vi "Autonomous Independent.vi"   [LabVIEW 2013]
doc: "This VI is called when autonomous begins, and will automatically be terminated when autonomous ends. You can carry out timed or sensor driven robot movement independently without needing to return to the caller."
uses:
  <vilib>/Rock Robotics/WPI/Solenoid/WPI_SolenoidValue.ctl
  Robot Global Data.vi
  <vilib>/Rock Robotics/WPI/Solenoid/WPI_SolenoidSetEnum.vi
  <vilib>/Rock Robotics/WPI/RobotDrive/WPI_RobotDriveArcadeDrive_Standard(NoSaturation).vi
  <vilib>/Rock Robotics/WPI/RobotDrive/WPI_RobotDriveGetSetRefNum.vi
  <vilib>/Rock Robotics/WPI/Joystick/WPI_JoystickGetSetRefNum.vi
panel:
  # "Be sure to right-click and choose Data Operations>>Make Current Value default if you want to save the array values with the VI"
types:
  T1 = typedef "WPI_JoystickDevRef.ctl" = cluster{"Device":T2}
  T2 = typedef "WPI_JoystickDeviceEnum.ctl" = enum16{"USB 1", "USB 2", "USB 3", "USB 4", "Kinect 1", "Kinect 2"}
  T3 = cluster{"axis 1 (x)":dbl, "axis 2 (y)":dbl, "axis 3 (throttle)":dbl, "axis 4":dbl, "axis 5":dbl, "axis 6":dbl}
  T4 = typedef "WPI_SolenoidValue.ctl" = enum16{"Off", "On", "Forward", "Reverse"}
  T5 = typedef "WPI_DigitalInputDevRef.ctl" = cluster{"DevStatus":errorcluster, "DIO Channel":T6, "Digital Module":T7}
  T6 = typedef "FPGA_DIOChannel.ctl" = enum8{"DIO 1", "DIO 2", "DIO 3", "DIO 4", "DIO 5", "DIO 6", "DIO 7", "DIO 8", "DIO 9", "DIO 10", "DIO 11", "DIO 12", "DIO 13", "DIO 14", "Invalid"}
  T7 = typedef "FPGA_TypedefDigitalModule.ctl" = enum16{"Digital Module 1", "Digital Module 2"}
  T8 = typedef "WPI_SolenoidDevRef.ctl" = cluster{"DevStatus":errorcluster, "Solenoid Module":T9, "Forward Solenoid Channel":T10, "Reverse Solenoid Channel":T10}
  T9 = typedef "FPGA_TypedefSolenoidModule.ctl" = enum16{"Solenoid Module 1", "Solenoid Module 2"}
  T10 = typedef "WPI_SolenoidChannel.ctl" = enum8{"Solenoid 1", "Solenoid 2", "Solenoid 3", "Solenoid 4", "Solenoid 5", "Solenoid 6", "Solenoid 7", "Solenoid 8", "Invalid"}
  T11 = typedef "WPI_RobotDriveDevRef.ctl" = cluster{"DevStatus":errorcluster, "Motors[]":T12[], "Square Inputs":bool, "Max Output":dbl, "Isochronous":bool}
  T12 = typedef "WPI_MotorControlDeviceRef.ctl" = cluster{"DeviceStatus":errorcluster, "Type":enum16{"PWM", "CAN"}, "PWM":cluster{"Digital Module":T7, "PWM Channel":T13, "DeadBand":T14}, "CAN":cluster{"Device Number":u8, "Control Mode":T15, "Semaphore":T16, "Max Vout":dbl}, "Invert":bool, "TransformRef":T17, "InvTransformRef":T17}
  T13 = typedef "FPGA_DIOPWMChannel.ctl" = enum8{"PWM 1", "PWM 2", "PWM 3", "PWM 4", "PWM 5", "PWM 6", "PWM 7", "PWM 8", "PWM 9", "PWM 10", "Invalid"}
  T14 = typedef "WPI_PWMDeadband.ctl" = cluster{"Name":string, "maxPositivePwm":i32, "minPositivePwm":i32, "centerPwm":i32, "maxNegativePwm":i32, "minNegativePwm":i32, "angularRange":u16}
  T15 = typedef "WPI_CANJaguar_ControlMode.ctl" = enum8{"Percent VBus", "Current", "Speed", "Position", "Voltage"}
  T16 = typedef "Semaphore RefNum" = refnum<k1>
  T17 = typedef "WPI_PWMTransform_ConPane.ctl" = refnum<vi>
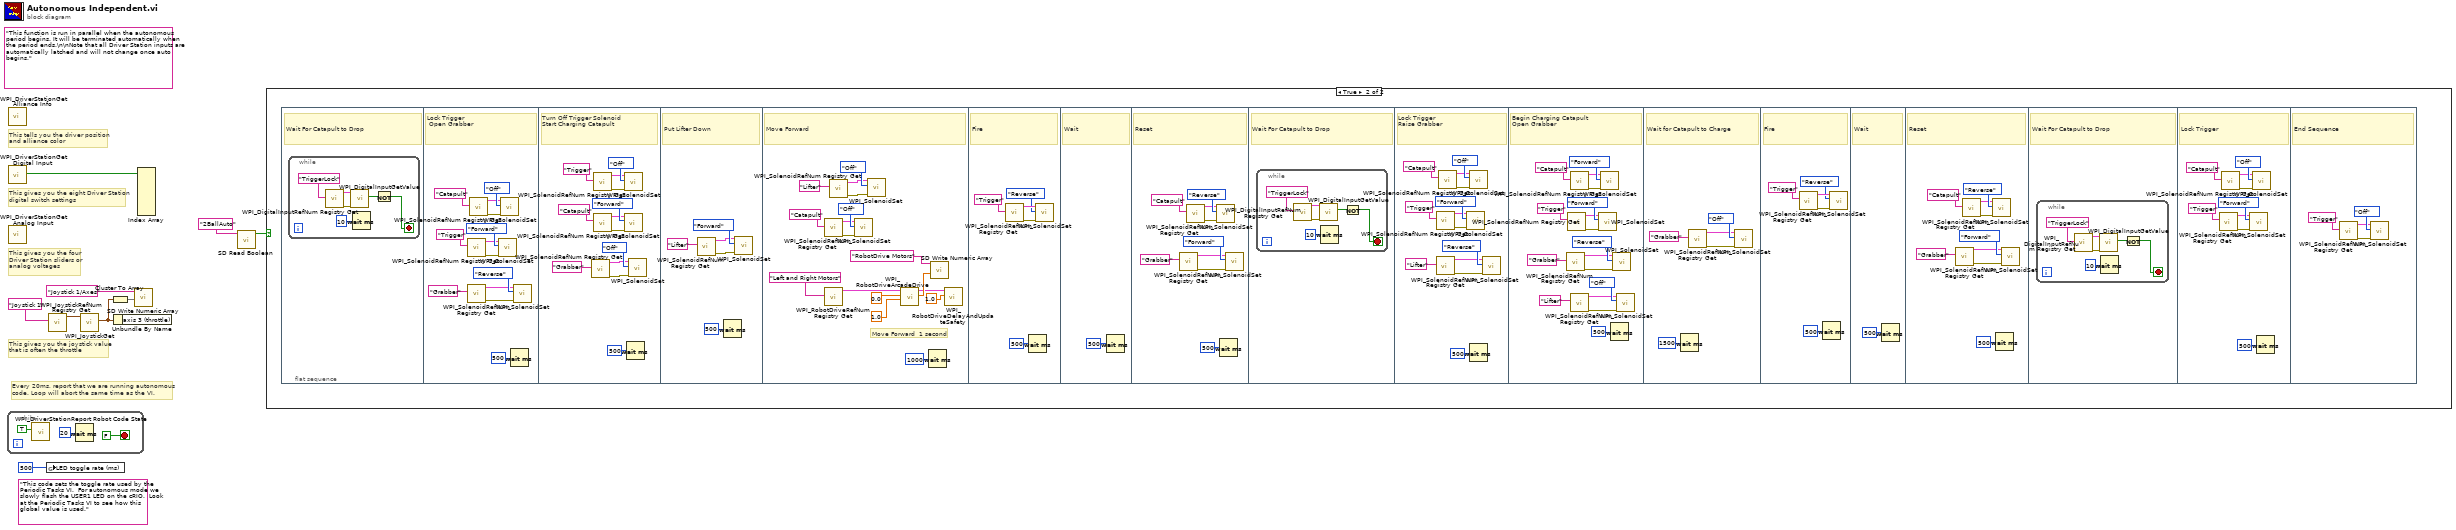
[diagram p0: block diagram]
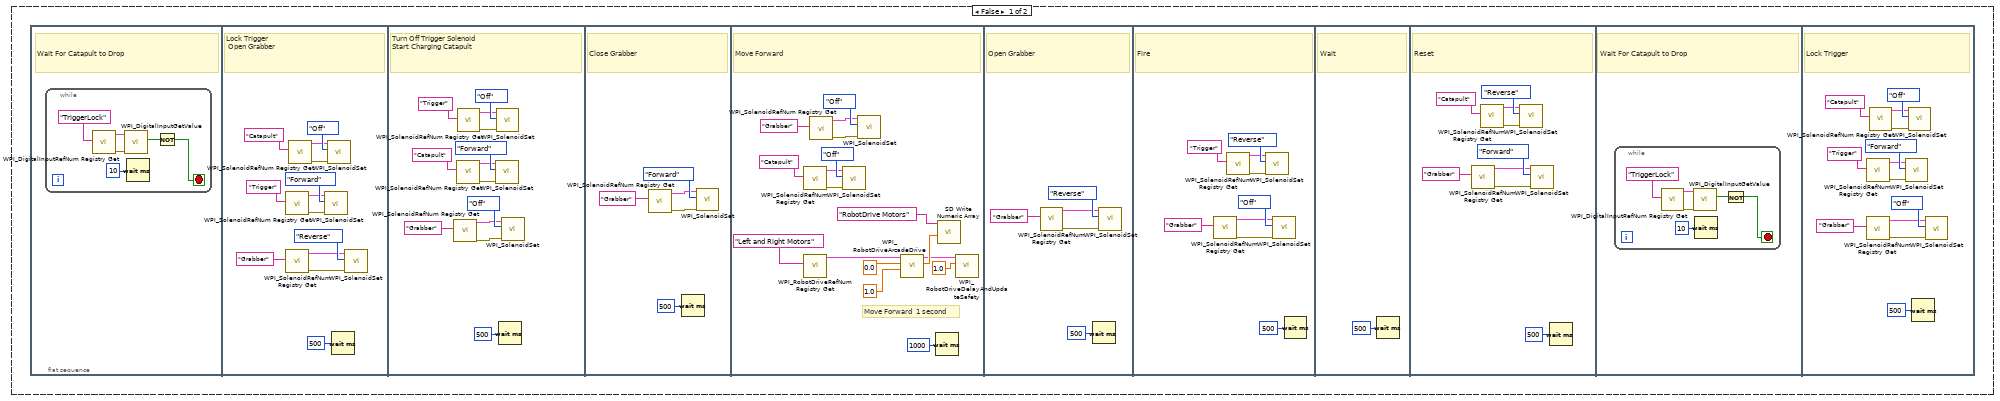
[diagram p2: hidden frame]
diagram:
  (unwired) "This code sets the toggle rate used by the Periodic Tasks VI.  For autonomous mode we slowly flash the USER1 LED on the cRIO.  Look at the Periodic Tasks VI to see how this global value is used."
  (unwired) "This function is run in parallel when the autonomous period begins. It will be terminated automatically when the period ends.\n\nNote that all Driver Station inputs are automatically latched and will not change once auto begins."
  # "Every 20ms, report that we are running autonomous\ncode. Loop will abort the same time as the VI."
  # "This gives you the joystick value\nthat is often the throttle"
  # "This tells you the driver position\nand alliance color"
  # "This gives you the eight Driver Station\ndigital switch settings"
  # "This gives you the four\nDriver Station sliders or\nanalog voltages"
  n1 = while {
    stop <- FALSE stop-if-true
    n2 = call <vilib>:"WPI_DriverStationReport Robot Code State.vi"("Autonomous"=TRUE) -> ()  [unwired: 10 in, 1 out]
    n3 = Wait (ms)(milliseconds to wait=u32 20) -> ()  [unwired: 1 out]
  }
  n4 = call <vilib>:"WPI_DriverStationGet Alliance Info.vi"() -> ()  [unwired: 12 out]
  n5 = call <vilib>:"WPI_DriverStationGet Digital Input.vi"() -> ("Driver Station Digital Input (1-8)"=w9:bool[])  [unwired: 11 out]
  n6 = call <vilib>:"WPI_DriverStationGet Analog Input.vi"() -> ()  [unwired: 12 out]
  n7 = global write "Robot Global Data.vi" "LED toggle rate (ms)"(u32 500 ("LED ms toggle rate")) -> ()
  n8 = call <vilib>:"WPI_JoystickRefNum Registry Get.vi"("refnum name"="Joystick 1") -> ("JoystickDevRef"=w7:T1)  [unwired: 1 in, 9 out]
  n9 = call <vilib>:"WPI_JoystickGet.vi"("JoystickDevRef"=w7) -> ("Axes"=w4:T3)  [unwired: 1 in, 5 out]
  n10 = Cluster To Array(cluster=w4) -> (array=w5:dbl[])
  n11 = Unbundle By Name(w4) -> ()  [unwired: 1 out]
  n12 = call <vilib>:"SD Write Numeric Array.vi"("Numeric Array"=w5, "Name"="Joystick 1/Axes") -> ()  [unwired: 8 in, 2 out]
  n13 = Index Array(array=w9) -> ()  [unwired: 8 in, 8 out]
  n14 = call <vilib>:"SD Read Boolean.vi"("Name"="2BallAuto") -> ("Boolean"=w1:bool)  [unwired: 8 in, 2 out]
  n15 = case shown="True" w1 {
    frame False {
      n16 = flat-sequence {
        frame #0 {
          # "Wait For Catapult to Drop"
          n17 = while {
            stop <- w14 stop-if-true
            n18 = call <vilib>:"WPI_DigitalInputRefNum Registry Get.vi"("refnum name"="TriggerLock") -> ("error out"=w15:errorcluster, "DigitalInputDevRef"=w16:T5)  [unwired: 9 in]
            n19 = call <vilib>:"WPI_DigitalInputGetValue.vi"("error in (no error)"=w15, "DigitalInputDevRef"=w16) -> ("Value"=w17:bool)  [unwired: 7 in, 2 out]
            n20 = Wait (ms)(milliseconds to wait=u32 10) -> ()  [unwired: 1 out]
            n21 = Not(x=w17) -> (.not. x?=w14:bool)
          }
        }
        frame #1 {
          # "Lock Trigger\n Open Grabber"
          n22 = call <vilib>:"WPI_SolenoidRefNum Registry Get.vi"("refnum name"="Trigger") -> ("error out"=w24:errorcluster, "SolenoidDevRef"=w25:T8)  [unwired: 9 in]
          n23 = call <vilib>:"WPI_SolenoidRefNum Registry Get.vi"("refnum name"="Grabber") -> ("error out"=w20:errorcluster, "SolenoidDevRef"=w21:T8)  [unwired: 9 in]
          n24 = call <vilib>:"WPI_SolenoidRefNum Registry Get.vi"("refnum name"="Catapult") -> ("error out"=w28:errorcluster, "SolenoidDevRef"=w29:T8)  [unwired: 9 in]
          n25 = call-poly <vilib>:"WPI_SolenoidSet.vi"("error in (no error)"=w24, "Value"=WPI_SolenoidValue."Forward", "SolenoidDevRef"=w25) -> ()  [unwired: 7 in, 2 out]
          n26 = call-poly <vilib>:"WPI_SolenoidSet.vi"("error in (no error)"=w28, "Value"=WPI_SolenoidValue."Off", "SolenoidDevRef"=w29) -> ()  [unwired: 7 in, 2 out]
          n27 = Wait (ms)(milliseconds to wait=u32 500) -> ()  [unwired: 1 out]
          n28 = call-poly <vilib>:"WPI_SolenoidSet.vi"("error in (no error)"=w20, "Value"=WPI_SolenoidValue."Reverse", "SolenoidDevRef"=w21) -> ()  [unwired: 7 in, 2 out]
        }
        frame #2 {
          # "Turn Off Trigger Solenoid\nStart Charging Catapult"
          n29 = call <vilib>:"WPI_SolenoidRefNum Registry Get.vi"("refnum name"="Grabber") -> ("error out"=w33:errorcluster, "SolenoidDevRef"=w34:T8)  [unwired: 9 in]
          n30 = call <vilib>:"WPI_SolenoidRefNum Registry Get.vi"("refnum name"="Catapult") -> ("error out"=w38:errorcluster, "SolenoidDevRef"=w39:T8)  [unwired: 9 in]
          n31 = call <vilib>:"WPI_SolenoidRefNum Registry Get.vi"("refnum name"="Trigger") -> ("error out"=w42:errorcluster, "SolenoidDevRef"=w43:T8)  [unwired: 9 in]
          n32 = call-poly <vilib>:"WPI_SolenoidSet.vi"("error in (no error)"=w38, "Value"=WPI_SolenoidValue."Forward", "SolenoidDevRef"=w39) -> ()  [unwired: 7 in, 2 out]
          n33 = call-poly <vilib>:"WPI_SolenoidSet.vi"("error in (no error)"=w42, "Value"=WPI_SolenoidValue."Off", "SolenoidDevRef"=w43) -> ()  [unwired: 7 in, 2 out]
          n34 = Wait (ms)(milliseconds to wait=u32 500) -> ()  [unwired: 1 out]
          n35 = call-poly <vilib>:"WPI_SolenoidSet.vi"("error in (no error)"=w33, "Value"=WPI_SolenoidValue."Off", "SolenoidDevRef"=w34) -> ()  [unwired: 7 in, 2 out]
        }
        frame #3 {
          # "Close Grabber"
          n36 = call <vilib>:"WPI_SolenoidRefNum Registry Get.vi"("refnum name"="Grabber") -> ("error out"=w46:errorcluster, "SolenoidDevRef"=w47:T8)  [unwired: 9 in]
          n37 = Wait (ms)(milliseconds to wait=u32 500) -> ()  [unwired: 1 out]
          n38 = call-poly <vilib>:"WPI_SolenoidSet.vi"("error in (no error)"=w46, "Value"=WPI_SolenoidValue."Forward", "SolenoidDevRef"=w47) -> ()  [unwired: 7 in, 2 out]
        }
        frame #4 {
          # "Move Forward  1 second"
          # "Move Forward"
          n39 = call <vilib>:"WPI_SolenoidRefNum Registry Get.vi"("refnum name"="Catapult") -> ("error out"=w51:errorcluster, "SolenoidDevRef"=w52:T8)  [unwired: 9 in]
          n40 = call <vilib>:"WPI_RobotDriveRefNum Registry Get.vi"("refnum name"="Left and Right Motors") -> ("RobotDriveDevRef"=w64:T11)  [unwired: 1 in, 9 out]
          n41 = call <vilib>:"WPI_SolenoidRefNum Registry Get.vi"("refnum name"="Grabber") -> ("error out"=w55:errorcluster, "SolenoidDevRef"=w56:T8)  [unwired: 9 in]
          n42 = call-poly <vilib>:"WPI_SolenoidSet.vi"("error in (no error)"=w51, "Value"=WPI_SolenoidValue."Off", "SolenoidDevRef"=w52) -> ()  [unwired: 7 in, 2 out]
          n43 = call-poly <vilib>:"WPI_SolenoidSet.vi"("error in (no error)"=w55, "Value"=WPI_SolenoidValue."Off", "SolenoidDevRef"=w56) -> ()  [unwired: 7 in, 2 out]
          n44 = call-poly <vilib>:"WPI_RobotDriveArcadeDrive.vi"("Y axis value"=1.0 ("X axis value"), "X axis value"=0.0, "RobotDriveDevRef"=w64) -> ("Motor Values"=w65:dbl[], "RobotDriveDevRef"=w61:T11)  [unwired: 1 in, 6 out]
          n45 = Wait (ms)(milliseconds to wait=u32 1000) -> ()  [unwired: 1 out]
          n46 = call <vilib>:"SD Write Numeric Array.vi"("Numeric Array"=w65, "Name"="RobotDrive Motors") -> ()  [unwired: 8 in, 2 out]
          n47 = call <vilib>:"WPI_RobotDriveDelayAndUpdateSafety.vi"("Delay (s)"=1.0, "RobotDriveDevRef"=w61) -> ()  [unwired: 8 in, 2 out]
        }
        frame #5 {
          # "Open Grabber"
          n48 = call <vilib>:"WPI_SolenoidRefNum Registry Get.vi"("refnum name"="Grabber") -> ("error out"=w69:errorcluster, "SolenoidDevRef"=w70:T8)  [unwired: 9 in]
          n49 = Wait (ms)(milliseconds to wait=u32 500) -> ()  [unwired: 1 out]
          n50 = call-poly <vilib>:"WPI_SolenoidSet.vi"("error in (no error)"=w69, "Value"=WPI_SolenoidValue."Reverse", "SolenoidDevRef"=w70) -> ()  [unwired: 7 in, 2 out]
        }
        frame #6 {
          # "Fire"
          n51 = call <vilib>:"WPI_SolenoidRefNum Registry Get.vi"("refnum name"="Grabber") -> ("error out"=w73:errorcluster, "SolenoidDevRef"=w74:T8)  [unwired: 9 in]
          n52 = call <vilib>:"WPI_SolenoidRefNum Registry Get.vi"("refnum name"="Trigger") -> ("error out"=w77:errorcluster, "SolenoidDevRef"=w78:T8)  [unwired: 9 in]
          n53 = call-poly <vilib>:"WPI_SolenoidSet.vi"("error in (no error)"=w77, "Value"=WPI_SolenoidValue."Reverse", "SolenoidDevRef"=w78) -> ()  [unwired: 7 in, 2 out]
          n54 = call-poly <vilib>:"WPI_SolenoidSet.vi"("error in (no error)"=w73, "Value"=WPI_SolenoidValue."Off", "SolenoidDevRef"=w74) -> ()  [unwired: 7 in, 2 out]
          n55 = Wait (ms)(milliseconds to wait=u32 500) -> ()  [unwired: 1 out]
        }
        frame #7 {
          # "Wait"
          n56 = Wait (ms)(milliseconds to wait=u32 500) -> ()  [unwired: 1 out]
        }
        frame #8 {
          # "Reset"
          n57 = call <vilib>:"WPI_SolenoidRefNum Registry Get.vi"("refnum name"="Grabber") -> ("error out"=w88:errorcluster, "SolenoidDevRef"=w89:T8)  [unwired: 9 in]
          n58 = call <vilib>:"WPI_SolenoidRefNum Registry Get.vi"("refnum name"="Catapult") -> ("error out"=w84:errorcluster, "SolenoidDevRef"=w85:T8)  [unwired: 9 in]
          n59 = call-poly <vilib>:"WPI_SolenoidSet.vi"("error in (no error)"=w84, "Value"=WPI_SolenoidValue."Reverse", "SolenoidDevRef"=w85) -> ()  [unwired: 7 in, 2 out]
          n60 = call-poly <vilib>:"WPI_SolenoidSet.vi"("error in (no error)"=w88, "Value"=WPI_SolenoidValue."Forward", "SolenoidDevRef"=w89) -> ()  [unwired: 7 in, 2 out]
          n61 = Wait (ms)(milliseconds to wait=u32 500) -> ()  [unwired: 1 out]
        }
        frame #9 {
          # "Wait For Catapult to Drop"
          n62 = while {
            stop <- w92 stop-if-true
            n63 = call <vilib>:"WPI_DigitalInputRefNum Registry Get.vi"("refnum name"="TriggerLock") -> ("error out"=w93:errorcluster, "DigitalInputDevRef"=w94:T5)  [unwired: 9 in]
            n64 = call <vilib>:"WPI_DigitalInputGetValue.vi"("error in (no error)"=w93, "DigitalInputDevRef"=w94) -> ("Value"=w95:bool)  [unwired: 7 in, 2 out]
            n65 = Wait (ms)(milliseconds to wait=u32 10) -> ()  [unwired: 1 out]
            n66 = Not(x=w95) -> (.not. x?=w92:bool)
          }
        }
        frame #10 {
          # "Lock Trigger"
          n67 = call <vilib>:"WPI_SolenoidRefNum Registry Get.vi"("refnum name"="Trigger") -> ("error out"=w102:errorcluster, "SolenoidDevRef"=w103:T8)  [unwired: 9 in]
          n68 = call <vilib>:"WPI_SolenoidRefNum Registry Get.vi"("refnum name"="Grabber") -> ("error out"=w98:errorcluster, "SolenoidDevRef"=w99:T8)  [unwired: 9 in]
          n69 = call <vilib>:"WPI_SolenoidRefNum Registry Get.vi"("refnum name"="Catapult") -> ("error out"=w106:errorcluster, "SolenoidDevRef"=w107:T8)  [unwired: 9 in]
          n70 = call-poly <vilib>:"WPI_SolenoidSet.vi"("error in (no error)"=w102, "Value"=WPI_SolenoidValue."Forward", "SolenoidDevRef"=w103) -> ()  [unwired: 7 in, 2 out]
          n71 = call-poly <vilib>:"WPI_SolenoidSet.vi"("error in (no error)"=w106, "Value"=WPI_SolenoidValue."Off", "SolenoidDevRef"=w107) -> ()  [unwired: 7 in, 2 out]
          n72 = Wait (ms)(milliseconds to wait=u32 500) -> ()  [unwired: 1 out]
          n73 = call-poly <vilib>:"WPI_SolenoidSet.vi"("error in (no error)"=w98, "Value"=WPI_SolenoidValue."Off", "SolenoidDevRef"=w99) -> ()  [unwired: 7 in, 2 out]
        }
      }
    }
    frame True {
      n74 = flat-sequence {
        frame #0 {
          # "Wait For Catapult to Drop"
          n75 = while {
            stop <- w111 stop-if-true
            n76 = call <vilib>:"WPI_DigitalInputRefNum Registry Get.vi"("refnum name"="TriggerLock") -> ("error out"=w112:errorcluster, "DigitalInputDevRef"=w113:T5)  [unwired: 9 in]
            n77 = call <vilib>:"WPI_DigitalInputGetValue.vi"("error in (no error)"=w112, "DigitalInputDevRef"=w113) -> ("Value"=w114:bool)  [unwired: 7 in, 2 out]
            n78 = Wait (ms)(milliseconds to wait=u32 10) -> ()  [unwired: 1 out]
            n79 = Not(x=w114) -> (.not. x?=w111:bool)
          }
        }
        frame #1 {
          # "Lock Trigger\n Open Grabber"
          n80 = call <vilib>:"WPI_SolenoidRefNum Registry Get.vi"("refnum name"="Trigger") -> ("error out"=w121:errorcluster, "SolenoidDevRef"=w122:T8)  [unwired: 9 in]
          n81 = call <vilib>:"WPI_SolenoidRefNum Registry Get.vi"("refnum name"="Grabber") -> ("error out"=w117:errorcluster, "SolenoidDevRef"=w118:T8)  [unwired: 9 in]
          n82 = call <vilib>:"WPI_SolenoidRefNum Registry Get.vi"("refnum name"="Catapult") -> ("error out"=w125:errorcluster, "SolenoidDevRef"=w126:T8)  [unwired: 9 in]
          n83 = call-poly <vilib>:"WPI_SolenoidSet.vi"("error in (no error)"=w121, "Value"=WPI_SolenoidValue."Forward", "SolenoidDevRef"=w122) -> ()  [unwired: 7 in, 2 out]
          n84 = call-poly <vilib>:"WPI_SolenoidSet.vi"("error in (no error)"=w125, "Value"=WPI_SolenoidValue."Off", "SolenoidDevRef"=w126) -> ()  [unwired: 7 in, 2 out]
          n85 = Wait (ms)(milliseconds to wait=u32 500) -> ()  [unwired: 1 out]
          n86 = call-poly <vilib>:"WPI_SolenoidSet.vi"("error in (no error)"=w117, "Value"=WPI_SolenoidValue."Reverse", "SolenoidDevRef"=w118) -> ()  [unwired: 7 in, 2 out]
        }
        frame #2 {
          # "Turn Off Trigger Solenoid\nStart Charging Catapult"
          n87 = call <vilib>:"WPI_SolenoidRefNum Registry Get.vi"("refnum name"="Grabber") -> ("error out"=w130:errorcluster, "SolenoidDevRef"=w131:T8)  [unwired: 9 in]
          n88 = call <vilib>:"WPI_SolenoidRefNum Registry Get.vi"("refnum name"="Catapult") -> ("error out"=w135:errorcluster, "SolenoidDevRef"=w136:T8)  [unwired: 9 in]
          n89 = call <vilib>:"WPI_SolenoidRefNum Registry Get.vi"("refnum name"="Trigger") -> ("error out"=w139:errorcluster, "SolenoidDevRef"=w140:T8)  [unwired: 9 in]
          n90 = call-poly <vilib>:"WPI_SolenoidSet.vi"("error in (no error)"=w135, "Value"=WPI_SolenoidValue."Forward", "SolenoidDevRef"=w136) -> ()  [unwired: 7 in, 2 out]
          n91 = call-poly <vilib>:"WPI_SolenoidSet.vi"("error in (no error)"=w139, "Value"=WPI_SolenoidValue."Off", "SolenoidDevRef"=w140) -> ()  [unwired: 7 in, 2 out]
          n92 = Wait (ms)(milliseconds to wait=u32 500) -> ()  [unwired: 1 out]
          n93 = call-poly <vilib>:"WPI_SolenoidSet.vi"("error in (no error)"=w130, "Value"=WPI_SolenoidValue."Off", "SolenoidDevRef"=w131) -> ()  [unwired: 7 in, 2 out]
        }
        frame #3 {
          # "Put Lifter Down"
          n94 = call <vilib>:"WPI_SolenoidRefNum Registry Get.vi"("refnum name"="Lifter") -> ("error out"=w143:errorcluster, "SolenoidDevRef"=w144:T8)  [unwired: 9 in]
          n95 = Wait (ms)(milliseconds to wait=u32 500) -> ()  [unwired: 1 out]
          n96 = call-poly <vilib>:"WPI_SolenoidSet.vi"("error in (no error)"=w143, "Value"=WPI_SolenoidValue."Forward", "SolenoidDevRef"=w144) -> ()  [unwired: 7 in, 2 out]
        }
        frame #4 {
          # "Move Forward  1 second"
          # "Move Forward"
          n97 = call <vilib>:"WPI_SolenoidRefNum Registry Get.vi"("refnum name"="Catapult") -> ("error out"=w148:errorcluster, "SolenoidDevRef"=w149:T8)  [unwired: 9 in]
          n98 = call <vilib>:"WPI_RobotDriveRefNum Registry Get.vi"("refnum name"="Left and Right Motors") -> ("RobotDriveDevRef"=w161:T11)  [unwired: 1 in, 9 out]
          n99 = call <vilib>:"WPI_SolenoidRefNum Registry Get.vi"("refnum name"="Lifter") -> ("error out"=w152:errorcluster, "SolenoidDevRef"=w153:T8)  [unwired: 9 in]
          n100 = call-poly <vilib>:"WPI_SolenoidSet.vi"("error in (no error)"=w148, "Value"=WPI_SolenoidValue."Off", "SolenoidDevRef"=w149) -> ()  [unwired: 7 in, 2 out]
          n101 = call-poly <vilib>:"WPI_SolenoidSet.vi"("error in (no error)"=w152, "Value"=WPI_SolenoidValue."Off", "SolenoidDevRef"=w153) -> ()  [unwired: 7 in, 2 out]
          n102 = call-poly <vilib>:"WPI_RobotDriveArcadeDrive.vi"("Y axis value"=1.0 ("X axis value"), "X axis value"=0.0, "RobotDriveDevRef"=w161) -> ("Motor Values"=w162:dbl[], "RobotDriveDevRef"=w158:T11)  [unwired: 1 in, 6 out]
          n103 = Wait (ms)(milliseconds to wait=u32 1000) -> ()  [unwired: 1 out]
          n104 = call <vilib>:"SD Write Numeric Array.vi"("Numeric Array"=w162, "Name"="RobotDrive Motors") -> ()  [unwired: 8 in, 2 out]
          n105 = call <vilib>:"WPI_RobotDriveDelayAndUpdateSafety.vi"("Delay (s)"=1.0, "RobotDriveDevRef"=w158) -> ()  [unwired: 8 in, 2 out]
        }
        frame #5 {
          # "Fire"
          n106 = call <vilib>:"WPI_SolenoidRefNum Registry Get.vi"("refnum name"="Trigger") -> ("error out"=w166:errorcluster, "SolenoidDevRef"=w165:T8)  [unwired: 9 in]
          n107 = Wait (ms)(milliseconds to wait=u32 500) -> ()  [unwired: 1 out]
          n108 = call-poly <vilib>:"WPI_SolenoidSet.vi"("error in (no error)"=w166, "Value"=WPI_SolenoidValue."Reverse", "SolenoidDevRef"=w165) -> ()  [unwired: 7 in, 2 out]
        }
        frame #6 {
          # "Wait"
          n109 = Wait (ms)(milliseconds to wait=u32 500) -> ()  [unwired: 1 out]
        }
        frame #7 {
          # "Reset"
          n110 = call <vilib>:"WPI_SolenoidRefNum Registry Get.vi"("refnum name"="Grabber") -> ("error out"=w175:errorcluster, "SolenoidDevRef"=w176:T8)  [unwired: 9 in]
          n111 = call <vilib>:"WPI_SolenoidRefNum Registry Get.vi"("refnum name"="Catapult") -> ("error out"=w171:errorcluster, "SolenoidDevRef"=w172:T8)  [unwired: 9 in]
          n112 = call-poly <vilib>:"WPI_SolenoidSet.vi"("error in (no error)"=w171, "Value"=WPI_SolenoidValue."Reverse", "SolenoidDevRef"=w172) -> ()  [unwired: 7 in, 2 out]
          n113 = Wait (ms)(milliseconds to wait=u32 500) -> ()  [unwired: 1 out]
          n114 = call-poly <vilib>:"WPI_SolenoidSet.vi"("error in (no error)"=w175, "Value"=WPI_SolenoidValue."Forward", "SolenoidDevRef"=w176) -> ()  [unwired: 7 in, 2 out]
        }
        frame #8 {
          # "Wait For Catapult to Drop"
          n115 = while {
            stop <- w180 stop-if-true
            n116 = call <vilib>:"WPI_DigitalInputRefNum Registry Get.vi"("refnum name"="TriggerLock") -> ("error out"=w181:errorcluster, "DigitalInputDevRef"=w182:T5)  [unwired: 9 in]
            n117 = call <vilib>:"WPI_DigitalInputGetValue.vi"("error in (no error)"=w181, "DigitalInputDevRef"=w182) -> ("Value"=w183:bool)  [unwired: 7 in, 2 out]
            n118 = Wait (ms)(milliseconds to wait=u32 10) -> ()  [unwired: 1 out]
            n119 = Not(x=w183) -> (.not. x?=w180:bool)
          }
        }
        frame #9 {
          # "Lock Trigger\nRaise Grabber"
          n120 = call <vilib>:"WPI_SolenoidRefNum Registry Get.vi"("refnum name"="Trigger") -> ("error out"=w191:errorcluster, "SolenoidDevRef"=w192:T8)  [unwired: 9 in]
          n121 = call <vilib>:"WPI_SolenoidRefNum Registry Get.vi"("refnum name"="Lifter") -> ("error out"=w187:errorcluster, "SolenoidDevRef"=w188:T8)  [unwired: 9 in]
          n122 = call <vilib>:"WPI_SolenoidRefNum Registry Get.vi"("refnum name"="Catapult") -> ("error out"=w195:errorcluster, "SolenoidDevRef"=w196:T8)  [unwired: 9 in]
          n123 = call-poly <vilib>:"WPI_SolenoidSet.vi"("error in (no error)"=w191, "Value"=WPI_SolenoidValue."Forward", "SolenoidDevRef"=w192) -> ()  [unwired: 7 in, 2 out]
          n124 = call-poly <vilib>:"WPI_SolenoidSet.vi"("error in (no error)"=w195, "Value"=WPI_SolenoidValue."Off", "SolenoidDevRef"=w196) -> ()  [unwired: 7 in, 2 out]
          n125 = Wait (ms)(milliseconds to wait=u32 500) -> ()  [unwired: 1 out]
          n126 = call-poly <vilib>:"WPI_SolenoidSet.vi"("error in (no error)"=w187, "Value"=WPI_SolenoidValue."Reverse", "SolenoidDevRef"=w188) -> ()  [unwired: 7 in, 2 out]
        }
        frame #10 {
          # "Begin Charging Catapult\nOpen Grabber"
          n127 = call <vilib>:"WPI_SolenoidRefNum Registry Get.vi"("refnum name"="Grabber") -> ("error out"=w203:errorcluster, "SolenoidDevRef"=w204:T8)  [unwired: 9 in]
          n128 = call <vilib>:"WPI_SolenoidRefNum Registry Get.vi"("refnum name"="Trigger") -> ("error out"=w207:errorcluster, "SolenoidDevRef"=w208:T8)  [unwired: 9 in]
          n129 = call <vilib>:"WPI_SolenoidRefNum Registry Get.vi"("refnum name"="Catapult") -> ("error out"=w211:errorcluster, "SolenoidDevRef"=w212:T8)  [unwired: 9 in]
          n130 = call <vilib>:"WPI_SolenoidRefNum Registry Get.vi"("refnum name"="Lifter") -> ("error out"=w199:errorcluster, "SolenoidDevRef"=w200:T8)  [unwired: 9 in]
          n131 = call-poly <vilib>:"WPI_SolenoidSet.vi"("error in (no error)"=w207, "Value"=WPI_SolenoidValue."Forward", "SolenoidDevRef"=w208) -> ()  [unwired: 7 in, 2 out]
          n132 = call-poly <vilib>:"WPI_SolenoidSet.vi"("error in (no error)"=w211, "Value"=WPI_SolenoidValue."Forward", "SolenoidDevRef"=w212) -> ()  [unwired: 7 in, 2 out]
          n133 = Wait (ms)(milliseconds to wait=u32 500) -> ()  [unwired: 1 out]
          n134 = call-poly <vilib>:"WPI_SolenoidSet.vi"("error in (no error)"=w203, "Value"=WPI_SolenoidValue."Reverse", "SolenoidDevRef"=w204) -> ()  [unwired: 7 in, 2 out]
          n135 = call-poly <vilib>:"WPI_SolenoidSet.vi"("error in (no error)"=w199, "Value"=WPI_SolenoidValue."Off", "SolenoidDevRef"=w200) -> ()  [unwired: 7 in, 2 out]
        }
        frame #11 {
          # "Wait for Catapult to Charge"
          n136 = Wait (ms)(milliseconds to wait=u32 1500) -> ()  [unwired: 1 out]
          n137 = call <vilib>:"WPI_SolenoidRefNum Registry Get.vi"("refnum name"="Grabber") -> ("error out"=w216:errorcluster, "SolenoidDevRef"=w217:T8)  [unwired: 9 in]
          n138 = call-poly <vilib>:"WPI_SolenoidSet.vi"("error in (no error)"=w216, "Value"=WPI_SolenoidValue."Off", "SolenoidDevRef"=w217) -> ()  [unwired: 7 in, 2 out]
        }
        frame #12 {
          # "Fire"
          n139 = call <vilib>:"WPI_SolenoidRefNum Registry Get.vi"("refnum name"="Trigger") -> ("error out"=w222:errorcluster, "SolenoidDevRef"=w221:T8)  [unwired: 9 in]
          n140 = Wait (ms)(milliseconds to wait=u32 500) -> ()  [unwired: 1 out]
          n141 = call-poly <vilib>:"WPI_SolenoidSet.vi"("error in (no error)"=w222, "Value"=WPI_SolenoidValue."Reverse", "SolenoidDevRef"=w221) -> ()  [unwired: 7 in, 2 out]
        }
        frame #13 {
          # "Wait"
          n142 = Wait (ms)(milliseconds to wait=u32 500) -> ()  [unwired: 1 out]
        }
        frame #14 {
          # "Reset"
          n143 = call <vilib>:"WPI_SolenoidRefNum Registry Get.vi"("refnum name"="Grabber") -> ("error out"=w231:errorcluster, "SolenoidDevRef"=w232:T8)  [unwired: 9 in]
          n144 = call <vilib>:"WPI_SolenoidRefNum Registry Get.vi"("refnum name"="Catapult") -> ("error out"=w227:errorcluster, "SolenoidDevRef"=w228:T8)  [unwired: 9 in]
          n145 = call-poly <vilib>:"WPI_SolenoidSet.vi"("error in (no error)"=w227, "Value"=WPI_SolenoidValue."Reverse", "SolenoidDevRef"=w228) -> ()  [unwired: 7 in, 2 out]
          n146 = Wait (ms)(milliseconds to wait=u32 500) -> ()  [unwired: 1 out]
          n147 = call-poly <vilib>:"WPI_SolenoidSet.vi"("error in (no error)"=w231, "Value"=WPI_SolenoidValue."Forward", "SolenoidDevRef"=w232) -> ()  [unwired: 7 in, 2 out]
        }
        frame #15 {
          # "Wait For Catapult to Drop"
          n148 = while {
            stop <- w236 stop-if-true
            n149 = call <vilib>:"WPI_DigitalInputRefNum Registry Get.vi"("refnum name"="TriggerLock") -> ("error out"=w237:errorcluster, "DigitalInputDevRef"=w238:T5)  [unwired: 9 in]
            n150 = call <vilib>:"WPI_DigitalInputGetValue.vi"("error in (no error)"=w237, "DigitalInputDevRef"=w238) -> ("Value"=w239:bool)  [unwired: 7 in, 2 out]
            n151 = Wait (ms)(milliseconds to wait=u32 10) -> ()  [unwired: 1 out]
            n152 = Not(x=w239) -> (.not. x?=w236:bool)
          }
        }
        frame #16 {
          # "Lock Trigger"
          n153 = call <vilib>:"WPI_SolenoidRefNum Registry Get.vi"("refnum name"="Trigger") -> ("error out"=w243:errorcluster, "SolenoidDevRef"=w244:T8)  [unwired: 9 in]
          n154 = call <vilib>:"WPI_SolenoidRefNum Registry Get.vi"("refnum name"="Catapult") -> ("error out"=w247:errorcluster, "SolenoidDevRef"=w248:T8)  [unwired: 9 in]
          n155 = call-poly <vilib>:"WPI_SolenoidSet.vi"("error in (no error)"=w243, "Value"=WPI_SolenoidValue."Forward", "SolenoidDevRef"=w244) -> ()  [unwired: 7 in, 2 out]
          n156 = call-poly <vilib>:"WPI_SolenoidSet.vi"("error in (no error)"=w247, "Value"=WPI_SolenoidValue."Off", "SolenoidDevRef"=w248) -> ()  [unwired: 7 in, 2 out]
          n157 = Wait (ms)(milliseconds to wait=u32 500) -> ()  [unwired: 1 out]
        }
        frame #17 {
          # "End Sequence"
          n158 = call <vilib>:"WPI_SolenoidRefNum Registry Get.vi"("refnum name"="Trigger") -> ("error out"=w251:errorcluster, "SolenoidDevRef"=w252:T8)  [unwired: 9 in]
          n159 = call-poly <vilib>:"WPI_SolenoidSet.vi"("error in (no error)"=w251, "Value"=WPI_SolenoidValue."Off", "SolenoidDevRef"=w252) -> ()  [unwired: 7 in, 2 out]
        }
      }
    }
  }
